vi "Init.vi"(8 "error in":errorcluster, 11 "VISA resource name":refnum<visa-resource-name>) -> (0 "error out":errorcluster, 3 "VISA resource name out":refnum<visa-resource-name>)   [LabVIEW 2014]
uses:
  <instrlib>/HMC-T2100/HMC-T2100.lvlib
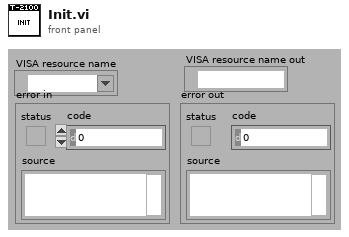
[diagram p1: front panel]
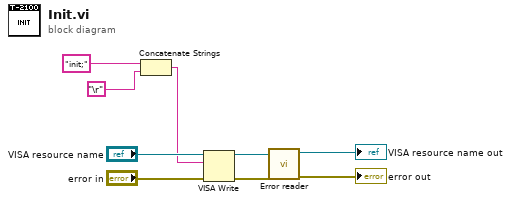
[diagram p0: block diagram]
diagram:
  n1 = Concatenate Strings("init;" ("write buffer"), "\r") -> (w5:string)
  n2 = VISA Write(VISA resource name="VISA resource name", write buffer=w5, error in (no error)="error in") -> (VISA resource name out=w3:refnum<visa-resource-name>, error out=w4:errorcluster)  [unwired: 1 out]
  n3 = call <instrlib>:"Error reader.vi"("error in"=w4, "T2100 Address In"=w3) -> ("error out"=→"error out":errorcluster, "T2100address Out"=→"VISA resource name out":refnum<visa-resource-name>)  [unwired: 8 out]
